vi "Main.vi"() -> ()   [LabVIEW 2013] (continued)
                w710 = TRUE ("Quit Flag")
                n449 = disable-structure shown="Disabled" {
                  frame Disabled {
                    n450 = call "Msgbox - Message Handler.vi"("<.?....> Message Code"="<W 104>") -> ("MHandler Error"=w711:errorcluster)  [unwired: 8 in, 2 out]
                    n451 = local write "MHandler"(w711) -> ()
                  }
                  frame Enabled {
                  }
                }
                n452 = local write "Quit Flag"(w710) -> ()
                n453 = property on="Stop Log off Event Structure" class="Bool (strict)"("Val(Sgnl)"=TRUE ("Value (Signaling)")) -> ()  [unwired: 2 in, 2 out]
              }
            }
          }
          frame True {
            # "Debug Close"
            n454 = flat-sequence {
              tunnel: [w715] -> w713
              frame #0 {
                w715 = TRUE ("T button?")
                n455 = local write "Quit Flag"(w715) -> ()
                n456 = property on="Stop Log off Event Structure" class="Bool (strict)"("Val(Sgnl)"=TRUE ("Value (Signaling)")) -> ()  [unwired: 2 in, 2 out]
              }
              frame #1 {
                n457 = Wait Until Next ms Multiple(millisecond multiple=u32 200) -> ()  [unwired: 1 out]
              }
              frame #2 {
                n458 = call "Queue - EnQueue to MessageQ.vi"("<NoD> Don't Display to UI"=TRUE, "Message"="{Debug CLOSE}" ("string")) -> ()  [unwired: 9 in, 1 out]
              }
            }
          }
        }
      }
      event Key Down? {
        # "44 Comma\n47 /\n92 \\"
        # "Disables comma in the entire program"
        n459 = event-data() -> ("Char"=w720:i16)  [unwired: 1 in, 9 out]
        n460 = case shown="44" w720 {
          tunnel: [_ w721 w722] -> w719
          frame 0, Default {
          }
          frame 47, 92 {
            w721 = TRUE  # Discard
            # "Discard all / and \\"
          }
          frame 44 {
            # "comma... \nReject if it is in Furnace Settings"
            n461 = local read "Master Data Tab"() -> (w726:enum32{"Material", "WPS", "Layout"})
            n462 = local read "Tab Setup"() -> (w728:enum32{"Part Details", "Furnace Settings"})
            n463 = Equal?(x=w728, y=enum32{"Part Details", "Furnace Settings"}."Furnace Settings") -> (x = y?=w723:bool)
            n464 = Equal?(x=w726, y=enum32{"Material", "WPS", "Layout"}."WPS") -> (x = y?=w724:bool)
            n465 = Or(x=w724, y=w723) -> (x .or. y?=w722:bool)
          }
        }
        n466 = event-data("Discard?"=w719) -> ()  [unwired: 1 in, 1 out]
      }
      event "------------------------------------        Setup TAB      ------------------------------------": Value Change {
        n467 = event-data() -> ()  [unwired: 1 in, 6 out]
      }
      event "Setup New", "Part Details Delete", "Setup New Toggle": Value Change {
        # "Reset TransactonNo, TransactionRunNo, Upload ET Flag"
        n468 = event-data() -> ("CtlRef"=w733:refnum<vi>)  [unwired: 1 in, 5 out]
        n469 = property class="Bool"(reference=w733) -> ("Label.Text"=w732:string)  [unwired: 1 in, 2 out]
        n470 = case shown="False" "Setup New Toggle" {
          tunnel: "Setup New" -> [w735 _]
          tunnel: [w734 TRUE ("OK Out")] -> w730
          frame False {
            # "Not From Logoff"
            n471 = case shown="True" w735 {
              tunnel: [TRUE ("OK Out") w746] -> w734
              frame False {
                w743 = 1  # Order No.
                # "Part Details Delete"
                n472 = property on="Part Details" class="MCListbox (strict)"() -> ("ItemNames"=w744:string[][], "Value"=w738:i32)  [unwired: 2 in, 2 out]
                n473 = Index Array(array=w744, index (row)=w738, index (col)=w743) -> (element=w740:string)
                n474 = call "Msgbox - Message Handler.vi"("Short Description (When DB Not Available)"="Part Details Deleted " ("string"), "Description (When DB Not Available)"=" details deleted." ("string"), "Pre-Description"=w740, "<.?....> Message Code"="<I 208>") -> ("MHandler Error"=w742:errorcluster)  [unwired: 5 in, 2 out]
                n475 = local write "MHandler"(w742) -> ()
              }
              frame True {
                # "Setup New"
                n476 = call "Msgbox - Message Handler.vi"("Short Description (When DB Not Available)"="Create New Setup", "Description (When DB Not Available)"="All unsaved data will be lost. Do you want to continue?", "<.?....> Message Code"="<W 201>") -> ("MHandler Error"=w749:errorcluster, "OK Out"=w746:bool)  [unwired: 6 in, 1 out]
                n477 = local write "MHandler"(w749) -> ()
              }
            }
          }
          frame True {
            # "Called From Logoff. No need to Prompt"
            n478 = local write "Setup New Toggle"(FALSE ("Setup New Toggle")) -> ()
          }
        }
        n479 = case shown="True" w730 {
          tunnel: w732 -> [_ w752]
          frame False {
          }
          frame True {
            n480 = case shown="\"Part Details Delete\"" w752 {
              tunnel: [_ w794] -> w753
              frame "Setup New", "Setup New Toggle", Default {
                w768 = 2 ("dimension size")
                w769 = 4 ("dimension size")
                n481 = flat-sequence {
                  frame #0 {
                    w778 = FALSE ("Visible")
                    w782 = "" ("Transaction No")
                    n482 = local write "Uploaded to ET"(FALSE ("Uploaded to ET")) -> ()
                    n483 = global write "Global SRTRS.vi" "[TransactionRunNo]"(w782) -> ()
                    n484 = local write "TransactionRunNo"(w782) -> ()
                    n485 = local write "TransactionRunNo (Execute)"(w782) -> ()
                    n486 = global write "Global SRTRS.vi" "[TransactionNo]"(w782) -> ()
                    n487 = local write "Transaction No (Execute)"(w782) -> ()
                    n488 = local write "Transaction No"(w782) -> ()
                    n489 = property on="TransactionRunNo" class="Str"("Visible"=w778) -> ()  [unwired: 2 in, 2 out]
                    n490 = property on="Transaction Details" class="Bool"("Visible"=w778) -> ()  [unwired: 2 in, 2 out]
                    n491 = property on="Setup Edit" class="Bool (strict)"("Value"=TRUE ("Setup Edit"), "DisabledEnum"=T30."Enabled" ("Disabled")) -> ()  [unwired: 2 in, 2 out]
                  }
                }
                n492 = control-ref of="MCListBox AWPS"() -> (w766:refnum<vi>)
                n493 = control-ref of="Extra Rev"() -> (w758:refnum<vi>)
                n494 = control-ref of="Additional WPS/Ref"() -> (w763:refnum<vi>)
                n495 = control-ref of="Extra WPS"() -> (w757:refnum<vi>)
                n496 = control-ref of="WPS Details Setup"() -> (w764:refnum<vi>)
                n497 = control-ref of="MCListBox FHS Setup"() -> (w767:refnum<vi>)
                n498 = control-ref of="Part Details"() -> (w777:refnum<vi>)
                n499 = Initialize Array("", w769) -> (w774:string[])
                n500 = Initialize Array("", w768) -> (w772:string[])
                n501 = invoke class="Str" method="Reinit To Default"(reference=w757) -> ()  [unwired: 2 in, 3 out]
                n502 = invoke class="Str" method="Reinit To Default"(reference=w758) -> ()  [unwired: 2 in, 3 out]
                n503 = invoke class="Clust (strict)" method="Reinit To Default"(reference=w764) -> ()  [unwired: 2 in, 3 out]
                n504 = invoke class="Clust (strict)" method="Reinit To Default"(reference=w763) -> ()  [unwired: 2 in, 3 out]
                n505 = Build Array(w774) -> (w773:string[][])
                n506 = Build Array(w772) -> (w771:string[][])
                n507 = property class="MCListbox (strict)"(reference=w777, "ItemNames"=string[][] [] ("Item Names")) -> ()  [unwired: 1 in, 2 out]
                n508 = property on="Property Node" class="MCListbox (strict)"(reference=w766, "ItemNames"=w771, "NumCols"=w768) -> (reference out=w765:refnum<vi>)  [unwired: 1 in, 1 out]
                n509 = property on="Property Node" class="MCListbox (strict)"(reference=w767, "ItemNames"=w773, "NumCols"=w769) -> (reference out=w756:refnum<vi>)  [unwired: 1 in, 1 out]
                n510 = disable-structure shown="Disabled" {
                  frame Disabled {
                    # "User not deleted"
                    n511 = control-ref of="User"() -> (w784:refnum<vi>)
                    n512 = invoke class="Str" method="Reinit To Default"(reference=w784) -> ()  [unwired: 2 in, 3 out]
                  }
                  frame Enabled {
                  }
                }
                n513 = flat-sequence {
                  frame #0 {
                    # "Only Default if NEW"
                    n514 = control-ref of="No."() -> (w783:refnum<vi>)
                    n515 = invoke class="DigNum (strict)" method="Reinit To Default"(reference=w783) -> ()  [unwired: 2 in, 3 out]
                  }
                }
                n516 = property on="Part Details Add" class="Bool (strict)"("DisabledEnum"=T30."Enabled" ("Disabled")) -> ()  [unwired: 2 in, 2 out]
                n517 = local read "CellBG Unused Cells"() -> (w762:u32)
                n518 = local read "Edit WPS in Setup"() -> (w755:bool)
                n519 = control-ref of="Tab Setup"() -> (w759:refnum<vi>)
                n520 = control-ref of="No."() -> (w754:refnum<vi>)
                n521 = call "MCListbox Refresh.vi"("color of New Cells"=w762, "color of Blank cells"=w762, "MulticolumnListbox in"=w756) -> ()  [unwired: 7 in, 2 out]
                n522 = call "MCListbox Refresh.vi"("color of New Cells"=w762, "color of Blank cells"=w762, "MulticolumnListbox in"=w765) -> ()  [unwired: 7 in, 2 out]
                n523 = call "Setup Tab - Enable-Disable.vi"("No."=w754, "MCListBox FHS Setup"=w756, "[SRTRS][Config][ParameterSettings] - [userEditableProcedure]"=w755, "Disabled"=T30."Enabled", "Tab Setup"=w759) -> ()  [unwired: 7 in]
              }
              frame "Part Details Delete" {
                # "Now No. is tied to Col0 value. So we can directly use Value."
                n524 = property on="Part Details" class="MCListbox (strict)"() -> ("ItemNames"=w787:string[][], "Value"=w786:i32)  [unwired: 2 in, 2 out]
                n525 = Delete From Array(array=w787, index (row)=w786) -> (array with subset deleted=w785:string[][])  [unwired: 2 in, 1 out]
                n526 = Array Size(array=w785) -> (size(s)=w792:i32[])
                n527 = Index Array(array=w792) -> (element=w791:i32)  [unwired: 1 in]
                n528 = for {
                  N: w791 -> [_]
                  tunnel: [w795] -> w790 mode=indexing
                  i -> [w796]
                  n529 = Increment(x=w796) -> (x+1=w795:i32)
                }
                n530 = Number To Decimal String(number=w790) -> (decimal integer string=w789:string[])  [unwired: 1 in]
                n531 = Replace Array Subset(array=w785, new element=w789, index (col)=0 ("disabled index (col)")) -> (w788:string[][])  [unwired: 1 in]
                n532 = property on="Part Details" class="MCListbox (strict)"("ItemNames"=w788) -> (error out=w794:errorcluster)  [unwired: 2 in, 1 out]
              }
            }
            n533 = flat-sequence {
              tunnel: w753 -> [_]
              frame #0 {
                # "Reset ALL to default after Delete or New Setup"
                n534 = control-ref of="Plot"() -> (w797:refnum<vi>)
                n535 = control-ref of="Setup Thermocouple Location"() -> (w799:refnum<vi>)
                n536 = control-ref of="Channel Mapping"() -> (w801:refnum<vi>)
                n537 = control-ref of="Notes"() -> (w800:refnum<vi>)
                n538 = control-ref of="Item Details"() -> (w802:refnum<vi>)
                n539 = invoke class="Str" method="Reinit To Default"(reference=w800) -> ()  [unwired: 2 in, 3 out]
                n540 = local write "Part Details"(-1 ("Part Details")) -> ()
                n541 = invoke class="Clust (strict)" method="Reinit To Default"(reference=w797) -> ()  [unwired: 2 in, 3 out]
                n542 = invoke class="Clust (strict)" method="Reinit To Default"(reference=w801) -> ()  [unwired: 2 in, 3 out]
                n543 = invoke class="Clust (strict)" method="Reinit To Default"(reference=w802) -> ()  [unwired: 2 in, 3 out]
                n544 = invoke class="Pict" method="Reinit To Default"(reference=w799) -> ()  [unwired: 2 in, 3 out]
              }
            }
          }
        }
      }
      event "Setup Save": Value Change {
        w807 = 19  # TC01Plot
        # "Check if any of the Plots are set to Plot"
        # "Wipe out the last row\nSolves the problem of having an incomplete last row"
        # "[1.2][2.4.1][“Save” Button]\nThe current setup is saved in a network shared folder (pre-defined in the\nconfiguration file) with the file name in the format of Transaction\nNumber_Date(YYYYMMDD)_Time(HHMMSS).stp.\nE.g. 0090312345_20130531_015020.stp"
        # "[1.2][2.4.1][Transaction Number]\nThis is a new running number automatically generated upon successful save\nof a process setup. This number will consist of 10 digits. First three digits will\nbe “009”, 4th and 5th digit will represent the furnace number, e.g. “03”, and\nthe last 5 digits will be the running number, e.g. 0090312345"
        n545 = event-data() -> ()  [unwired: 1 in, 1 out]
        n546 = Index Array "MCListBox Part Details"(array=w840, index=0) -> (element=w842:refnum<vi>)
        n547 = Index Array "MCListBox FHS Setup"(array=w840, index=1) -> (element=w839:refnum<vi>)
        n548 = property class="MCListbox (strict)"(reference=w839) -> (reference out=w833:refnum<vi>, "ItemNames"=w831:string[][])  [unwired: 1 in, 1 out]
        n549 = property class="MCListbox (strict)"(reference=w842) -> ("ItemNames"=w808:string[][])  [unwired: 1 in, 2 out]
        n550 = Array Size(array=w831) -> (size(s)=w838:i32[])
        n551 = Array Size(array=w808) -> (size(s)=w844:i32[])
        n552 = Index Array(array=w838) -> (element #1=w837:i32, element #2=w836:i32)  [unwired: 2 in]
        n553 = Array Subset(array=w808, index (col)=w807, length (col)=6 ("length")) -> (w805:string[][])  [unwired: 2 in]
        "TCxxPlots 2" <- w805
        n554 = Decrement(x=w837) -> (x-1=w832:i32)
        "FHS Last Row" <- w832
        n555 = for {
          tunnel: w805 -> [w848] mode=indexing
          tunnel: [w847] -> w804 mode=concatenating
          n556 = for {
            tunnel: w848 -> [w851] mode=indexing
            tunnel: [w849] -> w847 mode=indexing
            n557 = Equal?(x="1", y=w851) -> (x = y?=w849:bool)
          }
        }
        n558 = Initialize Array("", w836) -> (w834:string[])
        n559 = Index Array(array=w844, index=0) -> (element=w823:i32)
        n560 = Or Array Elements(Boolean array=w804) -> (logical OR=→"TCxxPlots":bool)
        n561 = Replace Array Subset(array=w831, new element=w834, index (row)=w832) -> (w829:string[][])  [unwired: 1 in]
        n562 = Greater Than 0?(x=w823) -> (x > 0?=w814:bool)
        "Part Details Complete" <- w814
        n563 = local read "WPS Details Setup"() -> (w828:T8)
        n564 = property class="MCListbox (strict)"(reference=w833, "ItemNames"=w829) -> (reference out=w824:refnum<vi>)  [unwired: 1 in, 1 out]
        n565 = Unbundle By Name(w828) -> ("Hold Temperature"=w827:string, "Hold Time (HH:MM)"=w826:string)
        n566 = call "String - Check Hold Parameters.vi"("Master Data Hold Time (HH:MM)"=w826, "Master Data Hold Temperature"=w827, "2D Array in"=w829) -> ("Found"=w813:bool)  [unwired: 6 in, 2 out]
        "FHS Hold Details Complete" <- w813
        n567 = call "String - Check Empty Cells.vi"("ItemNames"=w831) -> ("Empty Cell(s)"=w830:bool)  [unwired: 8 in, 2 out]
        n568 = Greater Than 0?(x=w832) -> (x > 0?=w816:bool)
        n569 = Not(x=w830) -> (.not. x?=w817:bool)
        n570 = And(x=w817, y=w816) -> (x .and. y?=w815:bool)
        "WPS Details Complete" <- w815
        n571 = property on="Output Set" class="CmbBox (strict)"() -> ("Value"=w819:T5)  [unwired: 2 in, 2 out]
        n572 = flat-sequence {
          tunnel: [w862] -> w821
          tunnel: [w854] -> w820
          tunnel: [w869] -> w809
          tunnel: [w868] -> w811
          frame #0 {
            w866 = 7  # Cal. Required
            (unwired) string[] ["Name", "Model", "Serial No.", "Last Cal. Date", "Next Cal. Due Date", "Equipment ID", "Notice Period", "Cal. Required"]  # 2015-01-01 11:16 ColHdr[]
            w873 = 5  # Equipment ID
            w880 = 6  # Notice Period
            w884 = 4  # Next Cal. Due Date
            # "Temperature Controller follows Furnace date"
            # "60 x 60 x 24 = 86,400 seconds/day"
            # "Check Calibration Date (Same Check done in {Recipe Start})"
            n573 = property on="Equipment Details" class="MCListbox (strict)"() -> ("ItemNames"=w872:string[][])  [unwired: 2 in, 2 out]
            n574 = property on="Next Calibration Due Date" class="Str"() -> ("Value"=w881:string)  [unwired: 2 in, 2 out]
            n575 = Array Size(array=w872) -> (size(s)=w871:i32[])
            n576 = Index Array(array=w871) -> (element=w870:i32)  [unwired: 1 in]
            n577 = Index Array(array=w872, index (col) #1=w884, index (col) #2=w880, index (col) #3=w873, index (col) #4=w866) -> (element #1=w852:string[], element #2=w853:string[], element #3=w879:string[], element #4=w865:string[])  [unwired: 4 in]
            n578 = Greater Than 0?(x=w870) -> (x > 0?=w868:bool)
            "Equipment Details Complete" <- w868
            n579 = Get Date/Time In Seconds() -> (seconds since 1Jan1904=w883:timestamp)
            n580 = call "DB - Convert BIT Type.vi"("BIT Type (eg Inactive) (Array)"=w865) -> ("Boolean (Array)"=w864:bool[])  [unwired: 2 in, 2 out]
            n581 = Build Array (concatenate)(w881, w852) -> ()  [unwired: 1 out]
            n582 = local read "Date Format (UserDefined)"() -> (w867:string)
            n583 = for {
              tunnel: w852 -> [w898] mode=indexing
              tunnel: w883 -> [w888]
              tunnel: [w892] -> w882 mode=indexing
              tunnel: w853 -> [w902] mode=indexing
              tunnel: w879 -> [w891] mode=indexing
              tunnel: [w891] -> w863 mode=indexing if=w899
              tunnel: w867 -> [w897]
              tunnel: w864 -> [w896] mode=indexing
              tunnel: [w891] -> w856 mode=indexing if=w890
              # "Next Cal Due Date - Today\n<= Notice Period"
              # "ALL FALSE will set Notice Due"
              n584 = Not(x=w896) -> (.not. x?=w894:bool)
              n585 = call "String - Convert UserDefined Date to SQL Date (YYYY-mm-dd).vi"("Date Format (UserDefined)"=w897, "Date String (UserDefined)"=w898) -> ("time stamp"=w889:timestamp)  [unwired: 7 in, 2 out]
              n586 = Decimal String To Number(string=w902) -> (number=w900:i32)  [unwired: 2 in, 1 out]
              n587 = Greater?(x=w889, y=w888) -> (0:w895:bool)
              n588 = Or(x=w895, y=w894) -> (x .or. y?=w892:bool)
              n589 = Multiply(x=86400.0, y=w900) -> (x*y=w886:dbl)
              n590 = Subtract(x=w889, y=w888) -> (x-y=w887:dbl)
              n591 = Less Or Equal?(x=w887, y=w886) -> (x <= y?=w885:bool)
              n592 = Compound Arithmetic op=OR "OR"(invert w892, invert w885, w894) -> (w893:bool)
              n593 = Not(x=w893) -> (.not. x?=w899:bool)
              n594 = Not(x=w892) -> (.not. x?=w890:bool)
            }
            "Calibration Date OK" <- w882
            n595 = And Array Elements(Boolean array=w882) -> (logical AND=w869:bool)
            "All Calibration Date Valid" <- w869
            n596 = Array To Spreadsheet String(delimiter (Tab)=",", array=w856, 3:"" ("format string")) -> (spreadsheet string=w860:string)
            n597 = Array To Spreadsheet String(delimiter (Tab)=",", array=w863, 3:"" ("format string")) -> (spreadsheet string=w875:string)
            n598 = Search and Replace String(replace all?=TRUE ("replace all? (F)"), input string=w860, search string="\r\n") -> (result string=→"Equipment ID Due List":string)  [unwired: 5 in, 3 out]
            n599 = Search and Replace String(replace all?=TRUE ("replace all? (F)"), input string=w875, search string="\r\n") -> (result string=w854:string)  [unwired: 5 in, 3 out]
            "Equipment ID Notice Due List" <- w854
            n600 = Empty Array?(array=w863) -> (empty?=w862:bool)
          }
        }
        n601 = Empty String/Path?(string/path=w819) -> (empty?=w818:bool)
        n602 = Not(x=w818) -> (.not. x?=w810:bool)
        "Output Set Details Complete" <- w810
        n603 = case shown="False" w821 {
          tunnel: w820 -> [w903 _]
          tunnel: [w906 TRUE ("OK Out")] -> w812
          frame False {
            # "At least one is less than xx Days"
            n604 = call "Msgbox - Message Handler.vi"("Short Description (When DB Not Available)"="Calibration Expiry Notification. " ("string"), "Description (When DB Not Available)"=" calibration validity expiring soon. Please arrange for calibration. Continue save?" ("string"), "Pre-Description"=w903, "<.?....> Message Code"="<W 212>") -> ("MHandler Error"=w908:errorcluster, "OK Out"=w906:bool)  [unwired: 5 in, 1 out]
            n605 = local write "MHandler"(w908) -> ()
          }
          frame True {
          }
        }
        n606 = Compound Arithmetic op=AND(w814, w815, w813, w812, w809, w811, w810) -> (w825:bool)
        n607 = case shown="True" w825 {
          tunnel: w840 -> [_ w1021]
          tunnel: w846 -> [_ w1024]
          tunnel: w824 -> [_ w1034]
          tunnel: w823 -> [_ w1016]
          tunnel: [_ w1015] -> w822
          frame False {
            # "6th  Check"
            # "5th  Check"
            # "4th  Check"
            # "2nd  Check (2)"
            # "2nd  Check (1)"
            # "1st Check"
            # "Not Valid"
            n608 = local read "Equipment Details Complete"() -> (w911:bool)
            n609 = local read "Output Set Details Complete"() -> (w910:bool)
            n610 = local read "FHS Hold Details Complete"() -> (w914:bool)
            n611 = local read "All Calibration Date Valid"() -> (w913:bool)
            n612 = local read "Part Details Complete"() -> (w916:bool)
            n613 = local read "WPS Details Complete"() -> (w915:bool)
            n614 = disable-structure shown="Disabled" {
              frame Disabled {
                (unwired) string[] ["Name", "Model", "Serial No.", "Last Cal. Date", "Next Cal. Due Date", "[EquipmentId]", "[NoticePeriod]"]  # 2014-11-18 16:27 Column Header Strings[]
                w924 = 2  # Serial No
                w923 = 1  # Model
                n615 = property on="Equipment Details" class="MCListbox (strict)"() -> ("ItemNames"=w922:string[][])  [unwired: 2 in, 2 out]
                n616 = Index Array(array=w922, index (col) #1=w923, index (col) #2=w924) -> (element #1=w926:string[], element #2=w928:string[])  [unwired: 2 in]
                n617 = local read "Calibration Date OK"() -> (w921:bool[])
                n618 = property on="Furnace Serial No" class="Str"() -> ("Value"=w927:string)  [unwired: 2 in, 2 out]
                n619 = Build Array (concatenate)("Furnace", w926) -> (w929:string[])
                n620 = Build Array (concatenate)(w927, w928) -> (w930:string[])
                n621 = for {
                  tunnel: w921 -> [w939] mode=indexing
                  tunnel: w929 -> [w938] mode=indexing
                  tunnel: w930 -> [w937] mode=indexing
                  shift-right: [w934] -> w932
                  shift-left: "" -> [w935]
                  i -> [w936]
                  n622 = case shown="False" w939 {
                    tunnel: w938 -> [w944 _]
                    tunnel: w937 -> [w945 _]
                    tunnel: w936 -> [_ _]
                    tunnel: w935 -> [w942 w949]
                    tunnel: [w946 w949] -> w934
                    frame False {
                      n623 = Empty String/Path?(string/path=w942) -> (empty?=w943:bool)
                      n624 = Select(t=w942, s=w943, f=", ") -> (s? t:f=w940:string)
                      n625 = Concatenate Strings(w942, w940, w944, " (Serial No: " ("string"), w945, ")" ("string")) -> (w946:string)
                    }
                    frame True {
                    }
                  }
                }
                n626 = Concatenate Strings(w932, " due for Calibration." ("string")) -> ()  [unwired: 1 out]
              }
              frame Enabled {
              }
            }
            n627 = case shown="True" w916 {
              tunnel: ["<E 210>" ("<.?....> Message Code") w959] -> w919
              tunnel: ["Add part details to proceed." ("<.?....> Message Code") w960] -> w918
              tunnel: w915 -> [_ w961]
              tunnel: w913 -> [_ w958]
              tunnel: ["No Part Details Found. " ("<.?....> Message Code") w957] -> w917
              tunnel: w914 -> [_ w956]
              tunnel: [_ w955] -> w912
              tunnel: w911 -> [_ w954]
              tunnel: w910 -> [_ w953]
              frame False {
                # "No Part Details Found"
              }
              frame True {
                # "Part Details Complete"
                n628 = case shown="True" w961 {
                  tunnel: ["Complete proper WPS Details to proceed." w970] -> w960
                  tunnel: ["<E 211>" w971] -> w959
                  tunnel: w958 -> [_ w972]
                  tunnel: ["WPS Details Incomplete." w969] -> w957
                  tunnel: w956 -> [_ w968]
                  tunnel: [_ w967] -> w955
                  tunnel: w954 -> [_ w966]
                  tunnel: w953 -> [_ w965]
                  frame False {
                    # "WPS contains incomplete OR insufficient Sequences"
                  }
                  frame True {
                    # "WPS Details Complete"
                    n629 = case shown="True" w968 {
                      tunnel: w972 -> [_ w979]
                      tunnel: ["<E 209>" w982] -> w971
                      tunnel: ["Hold. Temperature or Hold. Time does not match in Heating Sequence." w981] -> w970
                      tunnel: ["WPS Error" w980] -> w969
                      tunnel: [_ w978] -> w967
                      tunnel: w966 -> [_ w977]
                      tunnel: w965 -> [_ w976]
                      frame False {
                        # "FHS no matching Holding Temp or Time"
                      }
                      frame True {
                        # "FHS Hold Details Complete"
                        n630 = case shown="True" w979 {
                          tunnel: ["<E 213>" w991] -> w982
                          tunnel: [" calibration validity expired. Save Cancelled." w990] -> w981
                          tunnel: ["Calibration Expired" w989] -> w980
                          tunnel: [w984 _] -> w978
                          tunnel: w977 -> [_ w988]
                          tunnel: w976 -> [_ w987]
                          frame False {
                            # "Calibration Expired"
                            n631 = local read "Equipment ID Due List"() -> (w984:string)
                          }
                          frame True {
                            # "All Calibration Date Valid"
                            n632 = case shown="True" w988 {
                              tunnel: ["<E 214>" w995] -> w991
                              tunnel: ["Save Cancelled." w997] -> w990
                              tunnel: ["Equipment Not Available. " w996] -> w989
                              tunnel: w987 -> [_ w998]
                              frame False {
                                # "Equipment Not Available"
                              }
                              frame True {
                                # "Equipment Details Complete"
                                n633 = case shown="False" w998 {
                                tunnel: ["Please select a valid Output Set to proceed" _] -> w997
                                tunnel: ["Output Set Not Assigned" _] -> w996
                                tunnel: ["<E 215>" _] -> w995
                                frame False {
                                # "Output Set Details Incomplete"
                                }
                                frame True {
                                # "NA becasue all conditions \nare ANDed\nSo at least one would have failed"
                                # "Output Set Details Complete"
                                }
                                }
                              }
                            }
                          }
                        }
                      }
                    }
                  }
                }
              }
            }
            n634 = call "Msgbox - Message Handler.vi"("Short Description (When DB Not Available)"=w917, "Description (When DB Not Available)"=w918, "Pre-Description"=w912, "<.?....> Message Code"=w919) -> ("MHandler Error"=w920:errorcluster)  [unwired: 5 in, 2 out]
            n635 = local write "MHandler"(w920) -> ()
          }
          frame True {
            # "Log this entry 1st"
            # "All Cells Filled, MCListBox Part Details >0, MCListBox FHS Setup>0, Hold Parameters Valid"
            n636 = local read "DB - Setup Item (Part Details)"() -> (w1017:bool)
            n637 = local read "VISA resource name RS232"() -> (w1033:string)
            n638 = local read "WPS Details Setup"() -> (w1035:T8)
            n639 = case shown="False" w1017 {
              tunnel: [w1086 w1157] -> w1018
              tunnel: [w1124 _] -> w1014
              tunnel: [w1105 w1148] -> w1011
              tunnel: w1024 -> [w1102 _]
              tunnel: w1022 -> [w1088 _]
              tunnel: w1021 -> [w1087 _]
              frame False {
                w1094 = "Settings" ("section")
                # "Write Raw Strings will write \\ instead of \\\\"
                # "Create Transaction No"
                # "Update Running Number in ini file"
                # "Use File"
                n640 = local read "Furnace Number"() -> (w1122:string)
                n641 = local read "Running Number"() -> (w1119:i32)
                n642 = control-ref of="Parameter Buffer"() -> (w1101:refnum<vi>)
                n643 = Increment(x=w1119) -> (x+1=w1107:i32)
                n644 = Format Into String(format string="%05d", w1119) -> (resulting string=w1120:string)  [unwired: 2 in, 1 out]
                n645 = Format Date/Time String(time format string (%c)="%Y%m%d_%H%M%S") -> (date/time string=w1110:string)  [unwired: 2 in]
                n646 = Concatenate Strings("009" ("string"), w1122, w1120) -> (w1105:string)
                n647 = Build Array (concatenate)(w1102, w1101, w1088) -> (w1100:refnum<vi>[])
                n648 = Concatenate Strings(w1105, "_" ("string"), w1110, ".stp" ("string")) -> (w1129:string)
                n649 = call "Folder - Create Year-Month.vi"("Folder Name"="Setup") -> ("Folder with Year\\Month"=w1103:path)  [unwired: 9 in, 1 out]
                n650 = Build Path(base path=w1103, name or relative path=w1129) -> (appended path=w1092:path)
                n651 = call <vilib>:"Open Config Data.vi"("configuration file path"=w1092) -> ("error out"=w1127:errorcluster, "refnum"=w1128:T59)  [unwired: 8 in, 1 out]
                n652 = for {
                  tunnel: w1128 -> [w1140]
                  tunnel: w1127 -> [w1139]
                  tunnel: [w1138] -> w1125
                  tunnel: [w1137] -> w1126
                  tunnel: w1087 -> [w1136] mode=indexing
                  n653 = call "Key - MCListbox Write.vi"("error in (no error)"=w1139, "MulticolumnListbox Ref in"=w1136, "refnum"=w1140) -> ("error out"=w1137:errorcluster, "Refnum out"=w1138:T59)  [unwired: 5 in, 2 out]
                }
                n654 = for {
                  tunnel: w1100 -> [w1135] mode=indexing
                  tunnel: w1126 -> [w1134]
                  tunnel: w1125 -> [w1133]
                  tunnel: [w1132] -> w1090
                  tunnel: [w1131] -> w1089
                  n655 = call "Key - Cluster Write.vi"("error in (no error)"=w1134, "Cluster Ref in"=w1135, "Refnum in"=w1133) -> ("error out"=w1131:errorcluster, "Refnum out"=w1132:T59)  [unwired: 7 in]
                }
                n656 = local write "Latest stp file"(w1092) -> ()
                n657 = local write "Running Number"(w1107) -> ()
                n658 = call <vilib>:"Application Directory.vi"() -> ("Application Directory"=w1116:path)
                n659 = call <vilib>:"Close Config Data.vi"("error in (no error)"=w1089, "refnum"=w1090) -> ("file path"=w1124:path)  [unwired: 8 in, 1 out]
                n660 = Build Path(base path=w1116, name or relative path="SRTRS.ini" ("ini Name")) -> (appended path=w1114:path)
                n661 = Number To Decimal String(number=w1107) -> (decimal integer string=w1106:string)  [unwired: 1 in]
                n662 = call <vilib>:"Open Config Data.vi"("create file if necessary (T)"=FALSE, "configuration file path"=w1114) -> ("error out"=w1118:errorcluster, "refnum"=w1117:T59)  [unwired: 7 in, 1 out]
                n663 = Not A Number/Path/Refnum?(number/path/refnum=w1124) -> (NaN/Path/Refnum?=w1130:bool)
                n664 = Path To String(path=w1092) -> (string=w1093:string)
                n665 = call-poly <vilib>:"Write Key.vi"("section"=w1094, "error in (no error)"=w1118, "value"=w1106, "key"="Running Number", "refnum"=w1117) -> ("error out"=w1097:errorcluster, "refnum out"=w1099:T59)  [unwired: 4 in, 1 out]
                n666 = Not(x=w1130) -> (.not. x?=w1086:bool)
                n667 = call-poly <vilib>:"Write Key.vi"("write raw string? (F)"=TRUE, "section"=w1094, "error in (no error)"=w1097, "value"=w1093, "key"="Latest stp File", "refnum"=w1099) -> ("error out"=w1096:errorcluster, "refnum out"=w1098:T59)  [unwired: 3 in, 1 out]
                n668 = call <vilib>:"Close Config Data.vi"("error in (no error)"=w1096, "refnum"=w1098) -> ("error out"=w1085:errorcluster)  [unwired: 8 in, 1 out]
                n669 = local write "ini File Error"(w1085) -> ()
              }
              frame True {
                # "Only Needed for [Setup].[Header]"
                # "Blank [TransactionRunNo] for\nSRTRS.Setup.Header"
                # "No Error = Success (TRUE)"
                # "Use DB"
                n670 = local read "Transaction No"() -> (w1152:string)
                n671 = local read "DB Refnums II"() -> (w1141:T24)
                n672 = local read "DB Refnums"() -> (w1153:T23)
                n673 = Bundle("Transaction No"=w1152, "") -> (w1151:cluster{"Transaction No":string, string})  [unwired: 1 in]
                n674 = Build Array("SRTRS.Setup.Header" ("DB.Schema.Table")) -> (w1146:string[])
                n675 = call "DB - [Setup].[Item] (Part Details).vi"("DB - Setup Item Enum"=DB_-_Setup_Item_Enum."INSERT [Setup].[Header]", "DB.Schema.Table Array"=w1146, "Transaction"=w1151, "DB Refnums"=w1153, "DB Refnums II"=w1141) -> ("Transaction"=w1149:T19, "SUMMARY"=w1161:errorcluster)  [unwired: 5 in, 4 out]
                n676 = Build Array("SRTRS.Setup.Item" ("DB.Schema.Table")) -> (w1144:string[])
                n677 = call "DB - [Setup].[Item] (Part Details).vi"("DB - Setup Item Enum"=DB_-_Setup_Item_Enum."INSERT [Setup].[Item]", "DB.Schema.Table Array"=w1144, "Transaction"=w1149, "error in (no error)"=w1161, "DB Refnums"=w1153) -> ("SUMMARY"=w1155:errorcluster)  [unwired: 5 in, 5 out]
                n678 = Build Array("SRTRS.Setup.ProcedureItem" ("DB.Schema.Table")) -> (w1142:string[])
                n679 = call "DB - [Setup].[Item] (Part Details).vi"("DB - Setup Item Enum"=DB_-_Setup_Item_Enum."INSERT [Setup].[ProcedureItem]", "DB.Schema.Table Array"=w1142, "Transaction"=w1149, "error in (no error)"=w1155, "DB Refnums"=w1153) -> ("SUMMARY"=w1154:errorcluster)  [unwired: 5 in, 5 out]
                n680 = Unbundle By Name(w1149) -> ("TransactionNo"=w1148:string)
                n681 = Unbundle By Name(w1154) -> ("status"=w1158:bool)
                n682 = Not(x=w1158) -> (.not. x?=w1157:bool)
              }
            }
            n683 = local read "Simulate ET3500"() -> (w1032:bool)
            n684 = call "ET3500 - Write Program.vi"("Simulate"=w1032, "MCListBox FHS Setup"=w1034, "WPS Details Setup"=w1035, "VISA resource name RS232"=w1033) -> ("ET3500"=w1013:errorcluster, "Final Target Temperture"=w1023:i32, "Seq-Seg Info"=→"Seq-Seg Info":T17)  [unwired: 2 in, 3 out]
            n685 = flat-sequence {
              tunnel: w1023 -> [w1165]
              tunnel: [w1162] -> w1022
              frame #0 {
                # "We may be able to get Final Target Temperature for recovery\nif we Read the WPS Details Setup again."
                n686 = Number To Decimal String(number=w1165) -> (decimal integer string=w1164:string)  [unwired: 1 in]
                n687 = Bundle(w1164) -> (→"Final Target Temperature":cluster{string})  [unwired: 1 in]
                n688 = control-ref of="Final Target Temperature"() -> (w1162:refnum<vi>)
              }
            }
            n689 = local write "ET3500 Error"(w1013) -> ()
            n690 = case shown="Error" w1013 {
              tunnel: w1032 -> [w1192 _]
              tunnel: [TRUE FALSE] -> w1019
              frame No Error {
                n691 = Select(t="Simulate Upload to ET3504 OK." ("message"), s=w1192, f="Upload to ET3504 OK." ("message")) -> (s? t:f=w1186:string)
                n692 = Concatenate Strings("{Setup Save} ", w1186) -> (w1185:string)
                n693 = call "Queue - EnQueue to MessageQ.vi"("<NoD> Don't Display to UI"=TRUE, "Message"=w1185) -> ()  [unwired: 9 in, 1 out]
              }
              frame Error {
                (unwired) "Upload to ET3504 Failed. Check if ET3504 is already Running a Program. Check communication cable to ET3504." ("message")
                n694 = call "Msgbox - Message Handler.vi"("Short Description (When DB Not Available)"="Heating Sequence Upload Fail", "Description (When DB Not Available)"="Heating sequence program upload to furnace controller fail. Check the controller and retry", "<.?....> Message Code"="<E 220>") -> ("MHandler Error"=w1194:errorcluster)  [unwired: 6 in, 2 out]
                n695 = local write "MHandler"(w1194) -> ()
              }
            }
            n696 = Unbundle By Name("WPS Details Setup") -> ("WPS/Ref"=w1029:T5, "WPS Details Temperature Units"=w1030:string, "Hold Temperature"=w1031:string, "Hold Time (HH:MM)"=w1026:string)
            n697 = local write "Transaction No (Execute)"(w1011) -> ()
            n698 = local write "Transaction No"(w1011) -> ()
            n699 = global write "Global SRTRS.vi" "[TransactionNo]"(w1011) -> ()
            n700 = local write "Uploaded to ET"(w1019) -> ()
            n701 = local read "Info."() -> (w1027:T9)
            n702 = Bundle By Name(cluster=w1027, "Ref WPS"=w1029, "WPS"="Extra WPS", "Info. Temperature Units"=w1030, "Info. Temperature Units 2"=w1030, "Hold. Temp."=w1031, "Hold. Time (hour:minute)"=w1026) -> (w1025:T9)
            n703 = flat-sequence "SETUP TAB" {
              frame #0 {
                n704 = property on="Transaction Details" class="Bool"("Visible"=FALSE) -> ()  [unwired: 2 in, 2 out]
                n705 = property on="TransactionRunNo" class="Str"("Visible"=FALSE) -> ()  [unwired: 2 in, 2 out]
              }
            }
            n706 = local write "Info."(w1025) -> ()
            n707 = case shown="True" w1018 {
              frame False {
              }
              frame True {
                # "Save DB OR Save File OK"
                n708 = control-ref of="MCListBox FHS Setup"() -> (w1079:refnum<vi>)
                n709 = control-ref of="Tab Setup"() -> (w1082:refnum<vi>)
                n710 = local read "Edit WPS in Setup"() -> (w1081:bool)
                n711 = property on="Setup Edit" class="Bool (strict)"("DisabledEnum"=T30."Enabled" ("Disabled"), "Value"=FALSE ("Setup Edit")) -> ()  [unwired: 2 in, 2 out]
                n712 = control-ref of="No."() -> (w1078:refnum<vi>)
                n713 = call "Setup Tab - Enable-Disable.vi"("No."=w1078, "MCListBox FHS Setup"=w1079, "[SRTRS][Config][ParameterSettings] - [userEditableProcedure]"=w1081, "Disabled"=T30."Disabled", "Tab Setup"=w1082) -> ()  [unwired: 7 in]
              }
            }
            n714 = flat-sequence "EXECUTE TAB" {
              tunnel: w1025 -> [_]
              frame #0 {
                w1170 = FALSE ("Overall Status")
                w1171 = T36 [{"Color Box"=9868950, "Color Box 2"=9868950}, {"Color Box"=6618880, "Color Box 2"=6618880}, {"Color Box"=4934475, "Color Box 2"=4934475}, {"Color Box"=6618880, "Color Box 2"=6618880}]  # Init
                w1172 = T36 [{"Color Box"=9868950, "Color Box 2"=9868950}, {"Color Box"=6618880, "Color Box 2"=6618880}, {"Color Box"=4934475, "Color Box 2"=4934475}, {"Color Box"=6618880, "Color Box 2"=6618880}]  # Init
                w1173 = FALSE ("Value")
                w1168 = timestamp(3471350400 s since 1904-01-01) ("Parameter (Start Dwell Time)")
                # "Intialize"
                n715 = disable-structure shown="Disabled" {
                  frame Disabled {
                    n716 = invoke on="Chart" class="WFChart (strict)" method="Reinit To Default"() -> ()  [unwired: 3 in, 3 out]
                  }
                  frame Enabled {
                  }
                }
                n717 = local write "% Hold. Time Completed (Num)"(0.0 ("% Hold. Time Completed (Num)")) -> ()
                n718 = property on="Hold. Time (hour:minute)" class="Str"() -> ("Value"=w1177:string)  [unwired: 2 in, 2 out]
                n719 = local write "Parameter (End Dwell Time)"(w1168) -> ()
                n720 = local write "Parameter (Start Dwell Time)"(w1168) -> ()
                n721 = local write "Raw Data File"("") -> ()
                n722 = call "String - Format to (HH_colon_MM).vi"("xx:xx"=w1177) -> ("seconds"=w1178:dbl)  [unwired: 9 in, 1 out]
                n723 = property on="% Hold. Time Completed" class="Slide (strict)"("Scale.Maximum"=100.0 ("Scale.Range:Maximum"), "Scale.Minimum"=0.0 ("Scale.Range:Minimum"), "Fill Color"=u32 16777216 ("Color Box 2"), "Value"=0.0 ("% Hold Time Completed")) -> ()  [unwired: 2 in, 2 out]
                n724 = global read "Global SRTRS.vi" "Date Time Format"() -> (w1167:string)
                n725 = property on="Recording Duration" class="DigNum (strict)"("Value"=0.0) -> ()  [unwired: 2 in, 2 out]
                n726 = property on="Remaining Hold Time" class="DigNum (strict)"("Value"=w1178) -> ()  [unwired: 2 in, 2 out]
                n727 = property on="Variant Allowed (Hold Temp)" class="Bool (strict)"("Colors [4]"=w1172, "Value"=w1173) -> ()  [unwired: 2 in, 2 out]
                n728 = property on="Variant Allowed (Hold Time)" class="Bool (strict)"("Colors [4]"=w1172, "Value"=w1173) -> ()  [unwired: 2 in, 2 out]
                n729 = Format Date/Time String(time format string (%c)=w1167, seconds (now)=w1168) -> (date/time string=w1169:string)  [unwired: 1 in]
                n730 = Bundle By Name(cluster=T15 {"Start Holding Time and Date"="", "End Holding Time and Date"="", "Start Holding Temperature"="", "End Holding Temperature"=""} ("Parameter Buffer"), "Start Holding Time and Date"=w1169, "End Holding Time and Date"=w1169) -> (w1175:T15)
                n731 = property on="Hold Time Completed" class="Bool (strict)"("Colors [4]"=w1171, "Value"=w1170) -> ()  [unwired: 2 in, 2 out]
                n732 = property on="Process Completed" class="Bool (strict)"("Colors [4]"=w1171, "Value"=w1170) -> ()  [unwired: 2 in, 2 out]
                n733 = property on="Overall Status" class="Bool (strict)"("Colors [4]"=w1171, "Value"=w1170) -> ()  [unwired: 2 in, 2 out]
                n734 = local write "Parameter Buffer"(w1175) -> ()
                n735 = property on="Chart" class="WFChart (strict)"("History Data"=dynamicdata[] [[{"t0"=timestamp(3471350400 s since 1904-01-01), "dt"=1.0, "Y"=[0.0, 0.0]}]]) -> ()  [unwired: 2 in, 2 out]
              }
            }
            n736 = case shown="True" w1017 {
              tunnel: w1018 -> [w1047 w1065]
              tunnel: w1014 -> [w1040 _]
              tunnel: w1016 -> [w1049 w1067]
              tunnel: [w1048 w1066] -> w1015
              tunnel: w1011 -> [_ w1064]
              tunnel: [w1046 w1063] -> w1009
              tunnel: [w1045 w1062] -> w1008
              tunnel: [w1044 w1061] -> w1007
              tunnel: [w1038 w1060] -> w1003
              tunnel: [w1039 w1059] -> w1004
              frame False {
                w1042 = "\"" ("string")
                # "Use File"
                n737 = Path To String(path=w1040) -> (string=w1041:string)
                n738 = Concatenate Strings("FilePath: " ("string"), w1042, w1041, w1042) -> (w1038:string)
                n739 = case shown="True" w1047 {
                  tunnel: w1049 -> [_ w1058]
                  tunnel: [_ w1058] -> w1048
                  tunnel: ["<E 222>" ("<.?....> Message Code") "<I 221>" ("<.?....> Message Code")] -> w1046
                  tunnel: ["{Setup Save} Save File Failed." ("string") "{Setup Save} Save File" ("string")] -> w1039
                  tunnel: ["Setup Details Save Failed" ("Short Description (When DB Not Available)") "Setup Details Saved" ("Short Description (When DB Not Available)")] -> w1045
                  tunnel: ["Setup details not saved." ("<.?....> Message Code") "Setup details saved to Transaction number " ("Description (When DB Not Available)")] -> w1044
                  frame False {
                    # "File Save Not OK"
                  }
                  frame True {
                    # "File Save OK"
                  }
                }
              }
              frame True {
                # "Use DB"
                n740 = case shown="True" w1065 {
                  tunnel: w1067 -> [_ w1077]
                  tunnel: [_ w1077] -> w1066
                  tunnel: w1064 -> [_ w1073]
                  tunnel: ["<E 222>" ("<.?....> Message Code") "<I 221>" ("<.?....> Message Code")] -> w1063
                  tunnel: ["Setup Details Save Failed" ("Short Description (When DB Not Available)") "Setup Details Saved" ("Short Description (When DB Not Available)")] -> w1062
                  tunnel: ["Setup details not saved." ("<.?....> Message Code") "Setup details saved to Transaction number " ("Description (When DB Not Available)")] -> w1061
                  tunnel: [_ w1073] -> w1060
                  tunnel: ["{Setup Save} Insert DB Failed. [Setup].[Table]" ("string") "{Setup Save} Insert DB OK. [Setup].[Table}" ("string")] -> w1059
                  frame False {
                    # "Save  DB Failed"
                  }
                  frame True {
                    # "Save DB OK"
                  }
                }
              }
            }
            n741 = Concatenate Strings(w1004, w1003) -> (w1002:string)
            n742 = call "Queue - EnQueue to MessageQ.vi"("<NoD> Don't Display to UI"=TRUE, "Message"=w1002) -> ("Error Out"=w1005:errorcluster)  [unwired: 9 in]
            n743 = call "Msgbox - Message Handler.vi"("Short Description (When DB Not Available)"=w1008, "Description (When DB Not Available)"=w1007, "Error In (NA)"=w1005, "Post-Description"=w1003, "<.?....> Message Code"=w1009) -> ("MHandler Error"=w1010:errorcluster)  [unwired: 4 in, 2 out]
            n744 = local write "MHandler"(w1010) -> ()
          }
        }
        n745 = local write "No. of Items"(w822) -> ()
      }
      event "Setup Edit": Value Change {
        n746 = event-data() -> ()  [unwired: 1 in, 6 out]
        n747 = case shown="True" "Setup Edit" {
          selector: "Setup Edit" -> [w1210 _]
          tunnel: [TRUE ("OK Out") w1212] -> w1199
          tunnel: [w1210 w1212] -> w1198
          frame False {
          }
          frame True {
            n748 = call "Msgbox - Message Handler.vi"("Short Description (When DB Not Available)"="Edit Details Setup", "Description (When DB Not Available)"="Do you want to proceed to edit setup details?", "<.?....> Message Code"="<W 216>") -> ("MHandler Error"=w1215:errorcluster, "OK Out"=w1212:bool)  [unwired: 6 in, 1 out]
            n749 = local write "MHandler"(w1215) -> ()
          }
        }
        n750 = case shown="False" w1199 {
          tunnel: w1198 -> [_ w1202]
          frame False {
            # "Do not proceed.\nReset back to False"
            n751 = local write "Setup Edit"(FALSE ("Setup Edit")) -> ()
          }
          frame True {
            # "Procced to Enable/Disable"
            n752 = local read "Edit WPS in Setup"() -> (w1207:bool)
            n753 = control-ref of="MCListBox FHS Setup"() -> (w1208:refnum<vi>)
            n754 = control-ref of="Tab Setup"() -> (w1203:refnum<vi>)
            n755 = Select(t=T30."Enabled" ("Disabled"), s=w1202, f=T30."Disabled" ("Disabled")) -> (s? t:f=w1206:T30)
            n756 = control-ref of="No."() -> (w1209:refnum<vi>)
            n757 = call "Setup Tab - Enable-Disable.vi"("No."=w1209, "MCListBox FHS Setup"=w1208, "[SRTRS][Config][ParameterSettings] - [userEditableProcedure]"=w1207, "Disabled"=w1206, "Tab Setup"=w1203) -> ()  [unwired: 7 in]
          }
        }
      }
      event "Copy New": Value Change {
        # "Don't Display in UI AND\nDon't Log to MessageLog"
        n758 = event-data() -> ()  [unwired: 1 in, 6 out]
        n759 = call "Msgbox - Message Handler.vi"("Short Description (When DB Not Available)"="Copy Setup Details", "Description (When DB Not Available)"="Do you want to copy the current details to a new setup?", "<.?....> Message Code"="<W 217>") -> ("MHandler Error"=w1221:errorcluster, "OK Out"=w1219:bool)  [unwired: 6 in, 1 out]
        n760 = local write "MHandler"(w1221) -> ()
        n761 = case shown="True" w1219 {
          frame True {
            w1222 = FALSE ("Visible")
            w1223 = "" ("Transaction No")
            # "Same as Setup New"
            n762 = disable-structure shown="Disabled" {
              frame Disabled {
                # "Checked BY <Setup> Ready to Run for Blank TransactionNo"
                n763 = property on="Recipe Start" class="Bool"("DisabledEnum"=T30."Disabled and Grayed Out" ("Disabled")) -> ()  [unwired: 2 in, 2 out]
              }
              frame Enabled {
              }
            }
            n764 = global write "Global SRTRS.vi" "[TransactionRunNo]"(w1223) -> ()
            n765 = local write "TransactionRunNo"(w1223) -> ()
            n766 = local write "TransactionRunNo (Execute)"(w1223) -> ()
            n767 = global write "Global SRTRS.vi" "[TransactionNo]"(w1223) -> ()
            n768 = local write "Transaction No (Execute)"(w1223) -> ()
            n769 = local write "Transaction No"(w1223) -> ()
            n770 = local write "Uploaded to ET"(FALSE ("Uploaded to ET")) -> ()
            n771 = property on="TransactionRunNo" class="Str"("Visible"=w1222) -> ()  [unwired: 2 in, 2 out]
            n772 = property on="Transaction Details" class="Bool"("Visible"=w1222) -> ()  [unwired: 2 in, 2 out]
          }
          frame False {
          }
        }
      }
      event "Copy Setup", "Paste Setup": Value Change {
        n773 = event-data() -> ()  [unwired: 1 in, 6 out]
        n774 = Build Array("Copy Setup", "Paste Setup") -> (w1229:bool[])
        n775 = Search 1D Array(1D array=w1229, element=TRUE) -> (index of element=w1227:i32)  [unwired: 1 in]
        n776 = case shown="1" w1227 {
          tunnel: [w1232 w1237] -> w1226
          frame 0, Default {
            # "Copy"
            n777 = local read "DB Refnums"() -> (w1234:T23)
            n778 = call "Reference - Copy and Paste Buffer.vi"("Enum"=enum16{"Initialize", "Copy", "Paste"}."Copy", "DB Refnums"=w1234) -> ("error out"=w1232:errorcluster)  [unwired: 9 in]
            n779 = case shown="No Error" w1232 {
              frame No Error {
                n780 = property on="Paste Setup" class="Bool"("DisabledEnum"=T30."Enabled" ("Disabled")) -> ()  [unwired: 2 in, 2 out]
              }
              frame Error {
              }
            }
          }
          frame 1 {
            # "Paste"
            n781 = case shown="True" TRUE {
              tunnel: [_ w1238] -> w1237
              frame False {
              }
              frame True {
                n782 = local read "DB Refnums"() -> (w1240:T23)
                n783 = call "Reference - Copy and Paste Buffer.vi"("Enum"=enum16{"Initialize", "Copy", "Paste"}."Paste", "DB Refnums"=w1240) -> ("error out"=w1238:errorcluster)  [unwired: 9 in]
                n784 = flat-sequence {
                  frame #0 {
                    # "Reset ALL to default after delete"
                    n785 = control-ref of="Plot"() -> (w1241:refnum<vi>)
                    n786 = control-ref of="Notes"() -> (w1244:refnum<vi>)
                    n787 = control-ref of="Channel Mapping"() -> (w1245:refnum<vi>)
                    n788 = control-ref of="Setup Thermocouple Location"() -> (w1243:refnum<vi>)
                    n789 = control-ref of="Item Details"() -> (w1246:refnum<vi>)
                    n790 = local write "Part Details"(-1 ("Part Details")) -> ()
                    n791 = invoke class="Clust (strict)" method="Reinit To Default"(reference=w1241) -> ()  [unwired: 2 in, 3 out]
                    n792 = invoke class="Clust (strict)" method="Reinit To Default"(reference=w1245) -> ()  [unwired: 2 in, 3 out]
                    n793 = invoke class="Clust (strict)" method="Reinit To Default"(reference=w1246) -> ()  [unwired: 2 in, 3 out]
                    n794 = invoke class="Str" method="Reinit To Default"(reference=w1244) -> ()  [unwired: 2 in, 3 out]
                    n795 = invoke class="Pict" method="Reinit To Default"(reference=w1243) -> ()  [unwired: 2 in, 3 out]
                  }
                }
              }
            }
          }
        }
        "Copy/Paste DB Ref Nums" <- w1226
      }
      event "Search Setup": Value Change {
        n796 = event-data() -> ()  [unwired: 1 in, 6 out]
        n797 = flat-sequence {
          frame #0 {
            "From Search Button" <- TRUE ("From Search Button")
          }
          frame #1 {
            n798 = property on="Search Setup Toggle" class="Bool (strict)"() -> ("Value"=w1249:bool)  [unwired: 2 in, 2 out]
            n799 = Not(x=w1249) -> (.not. x?=w1248:bool)
            n800 = property on="Search Setup Toggle" class="Bool (strict)"("Val(Sgnl)"=w1248) -> ()  [unwired: 2 in, 2 out]
          }
        }
      }
      event "Search Setup Toggle": Value Change {
        # "Furnace Calibration and\nCompactRIO Module Details and\nInfo. (Execute Tab) (Variant Allowed for Temp and Time)\nnot overwritten here\nbecause they belong to the System."
        # "Load Setup Details from [Setup/Execute].[Header], [Setup/Execute].[Item], [Setup/Execute].[ProcedureItem]\nSet new [TransactionNo] and [TransactionRunNo]\nReset Uploaded to ET, Reset Setup Edit"
        n801 = event-data() -> ()  [unwired: 1 in, 6 out]
        n802 = local read "From Search Button"() -> (w1252:bool)
        n803 = local read "DB Refnums"() -> (w1251:T23)
        n804 = case shown="True" w1252 {
          tunnel: [w1292 w1335] -> w1253
          tunnel: w1251 -> [w1314 w1336]
          tunnel: [TRUE w1333] -> w1250
          frame False {
            w1309 = TRUE  # Simulate ET3500
            # "We just need the  Final Target Temperture\ncalculation, not going to DOWNLOAD program\nto ET3500"
            # "Event Fired from RecoveryFlag"
            n805 = global read "Global SRTRS.vi" "[TransactionNo]"() -> (w1312:string)
            n806 = global read "Global SRTRS.vi" "[TransactionRunNo]"() -> (w1313:string)
            n807 = Bundle("[TransactionNo]"=w1312, "[TransactionRunNo]"=w1313) -> (w1292:T60)  [unwired: 1 in]
            n808 = case shown="False" FALSE {
              tunnel: [w1327 w1329] -> w1315
              tunnel: [string[] ["SRTRS.Execute.Header", "SRTRS.Execute.Item", "SRTRS.MasterData.OutputSet"] string[] ["SRTRS.Setup.Header", "SRTRS.Setup.Item", "SRTRS.MasterData.OutputSet"]] -> w1316
              frame False {
                # "[TransactionRunNo] Exists\nUse SRTRS.Execute.*"
                n809 = Build Array("SRTRS.Execute.ProcedureItem" ("DB.Schema.Table")) -> (w1327:string[])
              }
              frame True {
                # "No [TransactionRunNo]\nUser SRTRS.Setup.*"
                n810 = Build Array("SRTRS.Setup.ProcedureItem" ("DB.Schema.Table")) -> (w1329:string[])
              }
            }
            n811 = call "DB - [Setup].[Item] (Part Details).vi"("DB - Setup Item Enum"=DB_-_Setup_Item_Enum."SELECT h.[TransactionNo], i.[OrderNo]", "DB.Schema.Table Array"=w1316, "Transaction"=w1292, "DB Refnums"=w1314) -> ()  [unwired: 6 in, 6 out]
